vi "Pre-lim Current Detection.vi"(6 "Barcodes in":string[](array[string]), 8 "error in (no error)":errorcluster, 11 "BoardHandle in 5":T1) -> (0 "Ch 4 High":dbl[](array[numeric]), 1 "Ch 3 High":dbl[](array[numeric]), 2 "Ch 2 High":dbl[](array[numeric]), 3 "Ch 1 High":dbl[](array[numeric]), 4 "error out":errorcluster, 5 "BoardHandle out 3":T1, 7 "Current High":bool)   [LabVIEW 2020]
uses:
  <instrlib>/CAEN PSM/CAEN PSM.lvlib
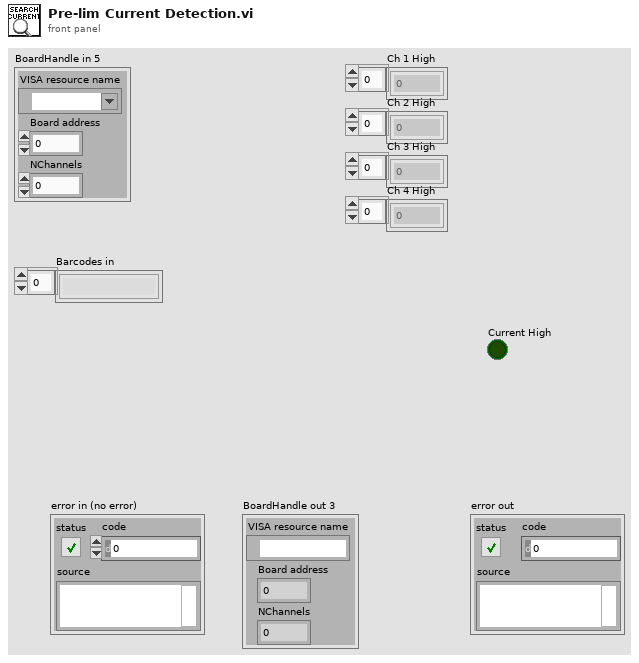
[diagram p1: front panel]
types:
  T1 = cluster{"VISA resource name":refnum<visa-resource-name>, "Board address":u8, "NChannels":u8}
  T2 = typedef "CAEN PSM.lvlib/BoardHandle.ctl" = cluster{"VISA resource name":refnum<visa-resource-name>, "Board address":i8, "NChannels":u8}
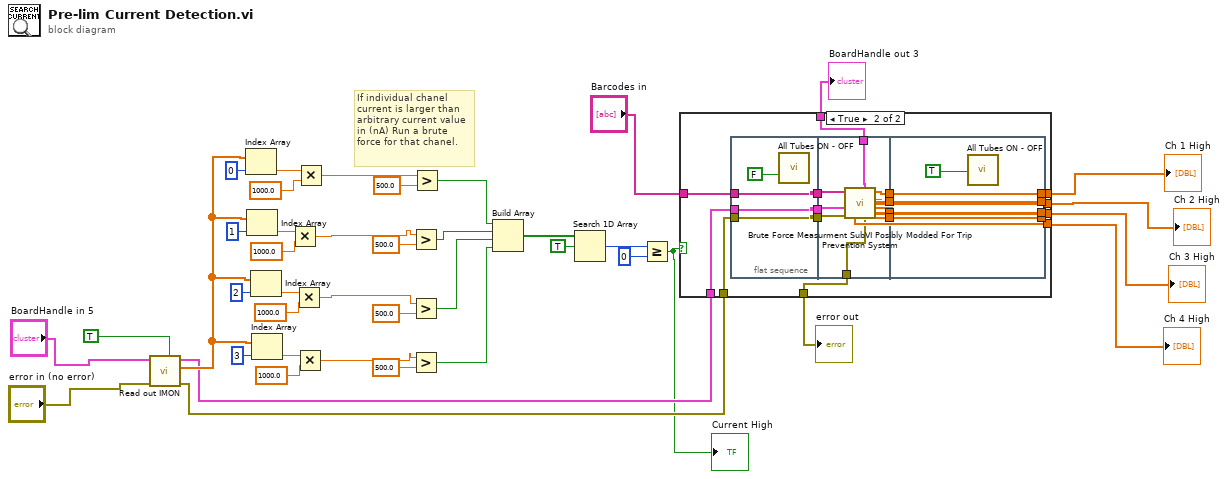
[diagram p0: block diagram]
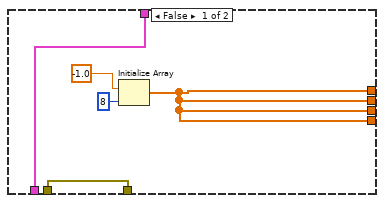
[diagram p2: hidden frame]
diagram:
  # "If individual chanel\ncurrent is larger than\narbitrary current value\nin (nA) Run a brute \nforce for that chanel."
  n1 = call <instrlib>:"Read out IMON.vi"("All Channels (T)"=TRUE ("All Channels (F)"), "error in (no error)"="error in (no error)", "BoardHandle"="BoardHandle in 5") -> ("error out"=w26:errorcluster, "IMon values (uA)"=w31:dbl[], "BoardHandle out"=w27:T2)  [unwired: 5 in, 1 out]
  n2 = Index Array(array=w31, index=0) -> (element=w30:dbl)
  n3 = Index Array(array=w31, index=1) -> (element=w40:dbl)
  n4 = Index Array(array=w31, index=2) -> (element=w37:dbl)
  n5 = Index Array(array=w31, index=3) -> (element=w34:dbl)
  n6 = Multiply(x=w40, y=1000.0) -> (x*y=w22:dbl)
  n7 = Multiply(x=w37, y=1000.0) -> (x*y=w21:dbl)
  n8 = Multiply(x=w34, y=1000.0) -> (x*y=w20:dbl)
  n9 = Multiply(x=w30, y=1000.0) -> (x*y=w29:dbl)
  n10 = Greater?(x=w22, y=500.0) -> (0:w18:bool)
  n11 = Greater?(x=w21, y=500.0) -> (0:w17:bool)
  n12 = Greater?(x=w20, y=500.0) -> (0:w16:bool)
  n13 = Greater?(x=w29, y=500.0) -> (0:w19:bool)
  n14 = Build Array(w19, w18, w17, w16) -> (w15:bool[])
  n15 = Search 1D Array(1D array=w15, element=TRUE) -> (index of element=w13:i32)  [unwired: 1 in]
  n16 = Greater Or Equal?(x=w13, y=0) -> (x >= y?=w11:bool)
  "Current High" <- w11
  n17 = case shown="True" w11 {
    tunnel: w27 -> [w47 w63]
    tunnel: w26 -> [w46 w62]
    tunnel: [w46 w61] -> w10
    tunnel: [w47 w60] -> w9
    tunnel: [w43 w59] -> w8
    tunnel: [w43 w58] -> w7
    tunnel: [w43 w57] -> w6
    tunnel: [w43 w56] -> w5
    tunnel: "Barcodes in" -> [_ w55]
    frame False {
      n18 = Initialize Array(-1.0, 8 ("dimension size")) -> (w43:dbl[])
    }
    frame True {
      n19 = flat-sequence {
        tunnel: w55 -> [w65]
        tunnel: w62 -> [w66]
        tunnel: w63 -> [w67]
        tunnel: [w67] -> w50
        tunnel: [w66] -> w49
        tunnel: [w65] -> w48
        tunnel: [w74] -> w61
        tunnel: [w73] -> w60
        tunnel: [w72] -> w54
        tunnel: [w71] -> w53
        tunnel: [w70] -> w52
        tunnel: [w69] -> w51
        tunnel: w50 -> [w76]
        tunnel: w49 -> [w75]
        tunnel: w48 -> [w68]
        tunnel: [w78] -> w56
        tunnel: [w79] -> w57
        tunnel: [w80] -> w58
        tunnel: [w81] -> w59
        tunnel: w54 -> [w81]
        tunnel: w53 -> [w80]
        tunnel: w52 -> [w79]
        tunnel: w51 -> [w78]
        frame #0 {
          n20 = call "All Tubes ON - OFF.vi"("Tubes ON/OFF"=FALSE) -> ()  [unwired: 11 in]
        }
        frame #1 {
          n21 = call "Brute Force Measurment SubVI Posibly Modded For Trip Prevention System.vi"("error in (no error)"=w75, "BoardHandle in"=w76, "Barcodes in"=w68) -> ("Ch 4 High"=w69:dbl[], "Ch 3 High"=w70:dbl[], "Ch 2 High"=w71:dbl[], "Ch 1 High"=w72:dbl[], "error out"=w74:errorcluster, "BoardHandle out"=w73:T1)  [unwired: 3 in]
        }
        frame #2 {
          n22 = call "All Tubes ON - OFF.vi"("Tubes ON/OFF"=TRUE) -> ()  [unwired: 11 in]
        }
      }
    }
  }
  "error out" <- w10
  "BoardHandle out 3" <- w9
  "Ch 1 High" <- w8
  "Ch 2 High" <- w7
  "Ch 3 High" <- w6
  "Ch 4 High" <- w5
